vi "Marker Or Cursor X And A B.vi"(0 "VISA resource name":refnum<visa-resource-name>, 1 "o - x Diff Marker Value (0,0)":dbl min=-9.99999e+37 max=9.99999e+37 format="%^.3e", 2 "LMark/oMark/LCurs(0:Line Curs)":u32(ring) items=["Line Cursor Value", "o Marker And Line Cur Diff value", "Line Cursor A", "Line Cursor B", "Line Cursor Average Point", "o Marker Position As Ref", "Width"], 3 "Line Curs Value (0,0)":dbl min=-9.99999e+37 max=9.99999e+37 format="%^.3e", 4 "o - L Diff Curs Value (0,0)":dbl min=-9.99999e+37 max=9.99999e+37 format="%^.3e", 5 "error in (no error)":errorcluster, 6 "o Ref-x Marker(T:o-x Diff val)":bool=TRUE, 7 "o And x Marker(0:o Marker Val)":u32(ring) items=["o Marker Value", "x Marker Value", "Store Sweep Range", "Partial Sweep Range On", "Partial Sweep Range Off", "o Marker Max A", "o Marker Min A", "o Marker Max B", "o Marker Min B", "Store Analysys Range", "Partial Analysis range On", "Partial Analysis Range Off"], 8 "o Marker Value (0,0)":dbl min=-9.99999e+37 max=9.99999e+37 format="%^.3e", 9 "o/x Marker Value (0,0)":dbl min=-9.99999e+37 max=9.99999e+37 format="%^.3e", 10 "o Marker (0:o Marker Value)":u32(ring) items=["o Marker Value", "o Marker Max of A", "o Marker Min of A", "o Marker Max of B", "o Marker Min of B"], 12 "Marker/LineCurs(1:oMarker On)":u32(ring)=1 items=["Marker And Line Cursor Off", "o Marker On", "o Reference - x Marker On", "o Line Marker On ", "o Marker And Line Cursor On ", "o Marker And x Marker On"]) -> (14 "VISA resource name out":refnum<visa-resource-name>, 19 "error out":errorcluster)   [LabVIEW 2017, in "Agilent 4194.lvlib"]
doc: "This function supports marker and cursor operations for mode X - A&B.\n\nNotes:\n\n(1) o is a sign for the first type of cursor/marker.\n\n(2) x is a sign for the second type of cursor/marker."
uses:
  Agilent 4194.lvlib
panel:
  # "o - x Diff Marker Value\no Marker Position As Ref"
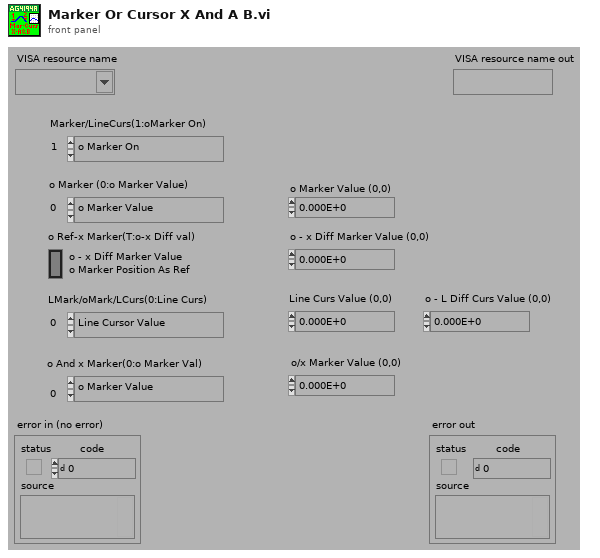
[diagram p1: front panel]
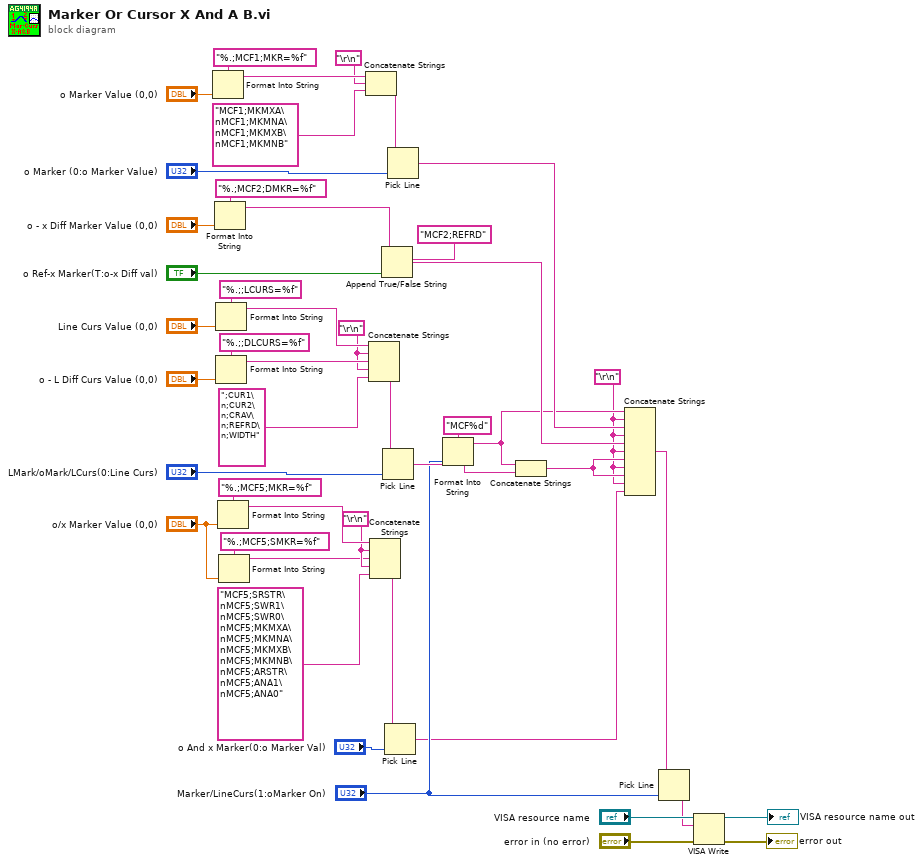
[diagram p0: block diagram]
diagram:
  w1 = "\r\n"
  w18 = "\r\n"
  w27 = "\r\n"
  n1 = Format Into String(format string="%.;MCF1;MKR=%f", "o Marker Value (0,0)") -> (resulting string=w44:string)  [unwired: 2 in, 1 out]
  n2 = Format Into String(format string="%.;MCF2;DMKR=%f", "o - x Diff Marker Value (0,0)") -> (resulting string=w36:string)  [unwired: 2 in, 1 out]
  n3 = Format Into String(format string="%.;;LCURS=%f", "Line Curs Value (0,0)") -> (resulting string=w33:string)  [unwired: 2 in, 1 out]
  n4 = Format Into String(format string="%.;;DLCURS=%f", "o - L Diff Curs Value (0,0)") -> (resulting string=w28:string)  [unwired: 2 in, 1 out]
  n5 = Format Into String(format string="%.;MCF5;MKR=%f", "o/x Marker Value (0,0)") -> (resulting string=w23:string)  [unwired: 2 in, 1 out]
  n6 = Format Into String(format string="%.;MCF5;SMKR=%f", "o/x Marker Value (0,0)") -> (resulting string=w17:string)  [unwired: 2 in, 1 out]
  n7 = Concatenate Strings(w44, "\r\n", "MCF1;MKMXA\nMCF1;MKMNA\nMCF1;MKMXB\nMCF1;MKMNB") -> (w40:string)
  n8 = Concatenate Strings(w33, w27, w28, w27, ";CUR1\n;CUR2\n;CRAV\n;REFRD\n;WIDTH") -> (w32:string)
  n9 = Concatenate Strings(w23, w18, w17, w18, "MCF5;SRSTR\nMCF5;SWR1\nMCF5;SWR0\nMCF5;MKMXA\nMCF5;MKMNA\nMCF5;MKMXB\nMCF5;MKMNB\nMCF5;ARSTR\nMCF5;ANA1\nMCF5;ANA0") -> (w22:string)
  n10 = Append True/False String(1:"o Ref-x Marker(T:o-x Diff val)", 2:"MCF2;REFRD", 3:w36) -> (0:w11:string)  [unwired: 1 in]
  n11 = Pick Line(multi-line string=w32, line index="LMark/oMark/LCurs(0:Line Curs)") -> (output string=w14:string)  [unwired: 1 in]
  n12 = Pick Line(multi-line string=w22, line index="o And x Marker(0:o Marker Val)") -> (output string=w3:string)  [unwired: 1 in]
  n13 = Pick Line(multi-line string=w40, line index="o Marker (0:o Marker Value)") -> (output string=w12:string)  [unwired: 1 in]
  n14 = Format Into String(format string="MCF%d", "Marker/LineCurs(1:oMarker On)") -> (resulting string=w4:string)  [unwired: 2 in, 1 out]
  n15 = Concatenate Strings(w4, w14) -> (w2:string)
  n16 = Concatenate Strings(w4, w1, w12, w1, w11, w1, w2, w1, w2, w1, w3) -> (w10:string)
  n17 = Pick Line(multi-line string=w10, line index="Marker/LineCurs(1:oMarker On)") -> (output string=w5:string)  [unwired: 1 in]
  n18 = VISA Write(VISA resource name="VISA resource name", write buffer=w5, error in (no error)="error in (no error)") -> (VISA resource name out=→"VISA resource name out":refnum<visa-resource-name>, error out=→"error out":errorcluster)  [unwired: 1 out]
